vi "Create Hard Links To Source.vi"(8 "Error In":errorcluster, 11 "Configuration":T1) -> (0 "Error Out":errorcluster, 3 "Configuration":T1)   [LabVIEW 2011, in "LVH-Build-Tools.lvlib"]
uses:
  <vilib>/LabVIEW Hacker/Build Tools/LVH-Build-Tools.lvlib
  Type Defs/Configuration.ctl
  Type Defs/Install Configuration.ctl
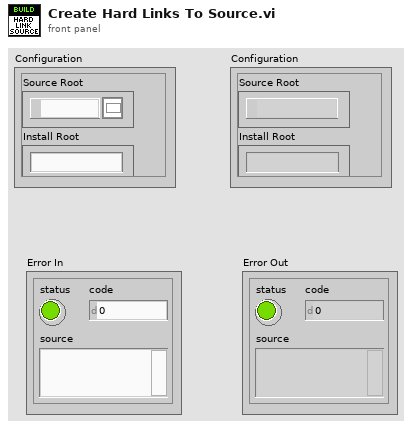
[diagram p1: front panel]
types:
  T1 = typedef "LVH-Build-Tools.lvlib/Configuration.ctl" = cluster{"Source Root":path, "Install Root":string, "Components":string[], "Ignore":string[], "Config Files":path[], "LV Directories":path[], "Install Paths":T2}
  T2 = typedef "LVH-Build-Tools.lvlib/Install Configuration.ctl" = cluster{"LabVIEW Directory":path, "Project Source Config":path}
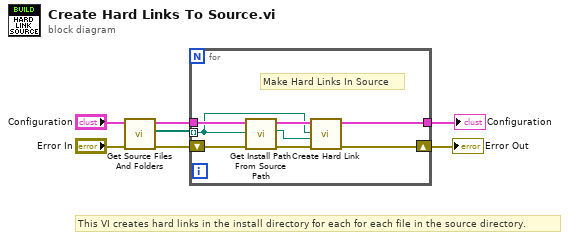
[diagram p0: block diagram]
diagram:
  # "This VI creates hard links in the install directory for each for each file in the source directory."
  n1 = call "Get Source Files And Folders.vi"("Error In"="Error In", "Configuration"="Configuration") -> ("Error Out"=w3:errorcluster, "All Source Files"=w1:path[], "Configuration"=w2:T1)  [unwired: 6 in, 1 out]
  n2 = for {
    shift-right: [w15] -> w7
    shift-left: w3 -> [w14]
    tunnel: w2 -> [w12]
    tunnel: w1 -> [w9] mode=indexing
    tunnel: [w10] -> w6
    # "Make Hard Links In Source"
    n3 = call "Get Install Path From Source Path.vi"("Error In"=w14, "Source File Path"=w9, "Configuration"=w12) -> ("Error Out"=w13:errorcluster, "Install File Path"=w8:path, "Configuration"=w11:T1)  [unwired: 5 in, 1 out]
    n4 = call "Create Hard Link.vi"("Error In"=w13, "Link Destination Path"=w8, "Existing File Path"=w9, "Configuration"=w11) -> ("Error Out"=w15:errorcluster, "Configuration"=w10:T1)  [unwired: 5 in, 1 out]
  }
  "Error Out" <- w7
  "Configuration" <- w6
